vi "CreateTDMSFileExample_ForDataExplorer.vi"() -> ()   [LabVIEW 2017]
uses:
  <vilib>/addons/InsightCM/Utilities/Tdms/Tdms.lvlib
  <vilib>/addons/InsightCM/Utilities/GlobalConfiguration/GlobalConfiguration.lvlib
  <vilib>/measure/NI_MABase.lvlib
  <vilib>/addons/InsightCM/Utilities/DeviceModelHelpers/DeviceModelHelpers.lvlib
panel:
  out "Created TDMS Files":path[](array[path])
  # "Run this VI and inspect the file(s) below"
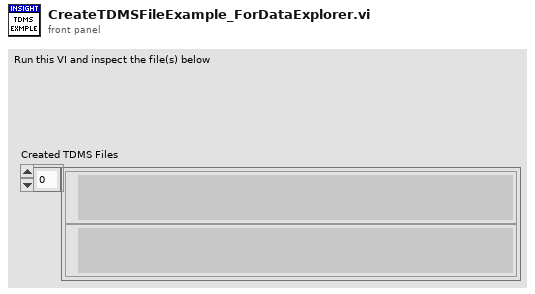
[diagram p1: front panel]
types:
  T1 = typedef "R2_DeviceModel.ctl" = cluster{"Device":T2, "Channels":T10[], "Tags":T12[]}
  T2 = typedef "R2_Device.ctl" = cluster{"Id":string, "Name":string, "DeviceType":string, "HardwareName":string, "IpAddress":string, "HardwareInfo":T3[], "ApplicationType":string, "ApplicationVersion":string, "EquipmentIds":string[], "ConfigurationVersion":string, "State":T4, "Properties":T3[], "DataGroups":T5[], "BurstModeTrigger":T9}
  T3 = typedef "KeyValuePair.ctl" = cluster{"Key":string, "Value":string}
  T4 = typedef "DeviceState.ctl" = cluster{"Disabled":bool}
  T5 = typedef "R2_DataGroup.ctl" = cluster{"Name":string, "OperatingStates":T6[], "Properties":T3[], "EquipmentIds":string[], "AssetNodeId":string}
  T6 = typedef "OperatingState.ctl" = cluster{"Name":string, "Properties":T3[], "Triggers":T7[]}
  T7 = typedef "Trigger.ctl" = cluster{"Type":string, "Expression":string, "Conditions":T8[]}
  T8 = typedef "Condition.ctl" = cluster{"Source":string, "Type":string, "Operator":string, "CompareTo":string, "DwellSeconds":dbl}
  T9 = typedef "BurstModeTrigger.ctl" = cluster{"Trigger":T7, "SampleRate":string, "AcquisitionLength":string}
  T10 = typedef "R2_Channel.ctl" = cluster{"Id":string, "DeviceId":string, "Name":string, "ChannelType":string, "HardwareKey":string, "HardwareChannel":string, "DataGroup":string, "Keywords":string[], "EquipmentIds":string[], "Properties":T3[], "Metrics":T11[], "AssetNodeId":string, "MeasType":string, "AssetName":string}
  T11 = typedef "Metric.ctl" = cluster{"Id":string, "Name":string, "Unit":string, "Properties":T3[], "MetricDefinitionInstanceId":string}
  T12 = typedef "Tag.ctl" = cluster{"Id":string, "Path":string, "Name":string, "Datatype":string, "Props":T3[], "Keywords":string[]}
  T13 = typedef "Equipment.ctl" = cluster{"Id":string, "ParentId":string, "Levelname":string, "Name":string, "Properties":T3[]}
  T14 = enum16{"open", "open or create", "create or replace", "create", "open (read-only)"}
  T15 = typedef "Tdms.lvlib/Property.ctl" = cluster{"Name":string, "Value":variant}
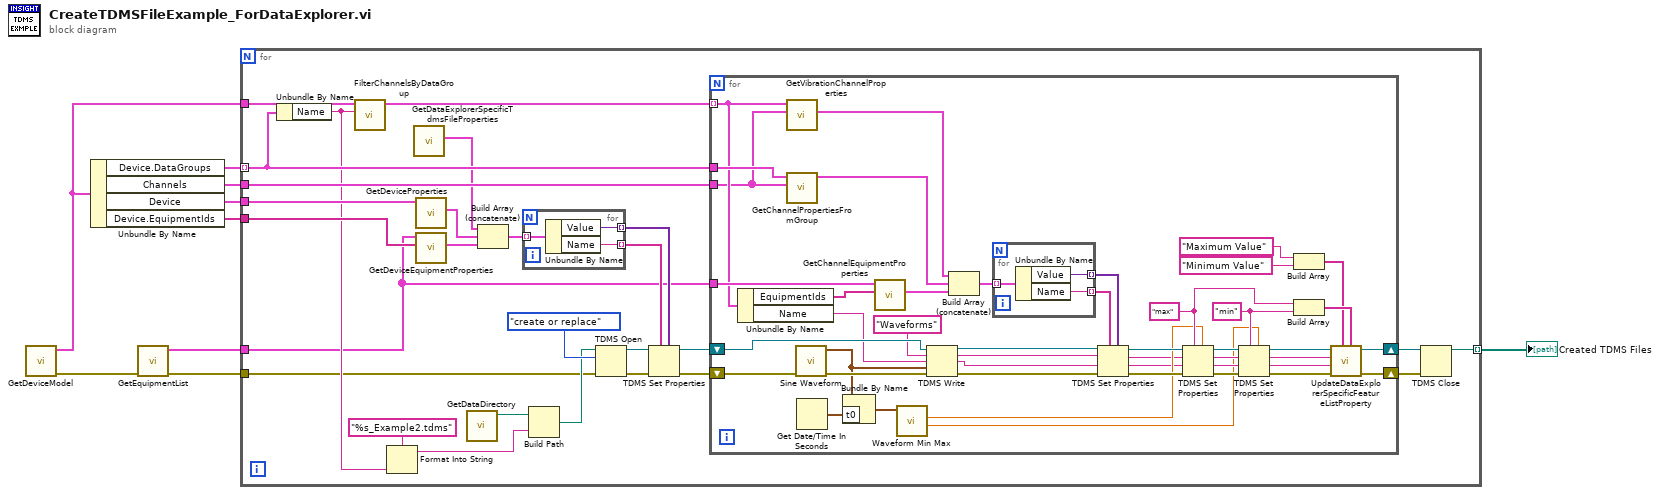
[diagram p0: block diagram]
diagram:
  n1 = call <vilib>:"GetDeviceModel.vi"() -> ("error out"=w3:errorcluster, "device model"=w5:T1)  [unwired: 9 in, 1 out]
  n2 = Unbundle By Name(w5) -> ("Device.DataGroups"=w6:T5[], "Channels"=w7:T10[], "Device"=w9:T2, "Device.EquipmentIds"=w8:string[])
  n3 = call <vilib>:"GetEquipmentList.vi"("error in (no error)"=w3) -> ("error out"=w2:errorcluster, "equipment list"=w1:T13[])  [unwired: 8 in, 1 out]
  n4 = for {
    tunnel: w2 -> [w11]
    tunnel: w9 -> [w36]
    tunnel: w8 -> [w35]
    tunnel: w7 -> [w21]
    tunnel: w6 -> [w17] mode=indexing
    tunnel: w5 -> [w19]
    tunnel: [w13] -> w4 mode=indexing
    tunnel: w1 -> [w10]
    n5 = Unbundle By Name(w17) -> ("Name"=w15:string)
    n6 = call <vilib>:"FilterChannelsByDataGroup.vi"("group"=w15, "device model"=w19) -> ("channels in data group"=w20:T10[])  [unwired: 8 in, 1 out]
    n7 = Format Into String(format string="%s_Example2.tdms", w15) -> (resulting string=w14:string)  [unwired: 2 in, 1 out]
    n8 = call <vilib>:"GetDataExplorerSpecificTdmsFileProperties.vi"() -> ("TDMS properties"=w12:T15[])  [unwired: 10 in, 1 out]
    n9 = call <vilib>:"GetDeviceProperties.vi"("device"=w36) -> ("tdms properties"=w31:T15[])  [unwired: 10 in]
    n10 = call <vilib>:"GetDeviceEquipmentProperties.vi"("equipment Ids"=w35, "equipment list"=w10) -> ("tdms properties"=w30:T15[])  [unwired: 9 in]
    n11 = call <vilib>:"GetDataDirectory.vi"() -> ("data directory"=w22:path)  [unwired: 10 in, 1 out]
    n12 = Build Array (concatenate)(w12, w31, w30) -> (w29:T15[])
    n13 = for {
      tunnel: w29 -> [w87] mode=indexing
      tunnel: [w86] -> w28 mode=indexing
      tunnel: [w85] -> w27 mode=indexing
      n14 = Unbundle By Name(w87) -> ("Value"=w85:variant, "Name"=w86:string)
    }
    n15 = Build Path(base path=w22, name or relative path=w14) -> (appended path=w18:path)
    n16 = TDMS Open(8:w11, 10:T14."create or replace" ("operation (0:open)"), 11:w18) -> (0:w32:errorcluster, 3:w33:refnum<k34>)  [unwired: 4 in]
    n17 = TDMS Set Properties(5:w27, 7:w28, 8:w32, 11:w33) -> (0:w26:errorcluster, 3:w25:refnum<k34>)  [unwired: 2 in, 2 out]
    n18 = for {
      shift-right: [w46] -> w23
      shift-left: w26 -> [w72]
      tunnel: w21 -> [w64]
      tunnel: w10 -> [w80]
      shift-right: [w45] -> w24
      shift-left: w25 -> [w74]
      tunnel: w20 -> [w65] mode=indexing
      tunnel: w17 -> [w66]
      w52 = "min" ("property names")
      w53 = "max" ("property names")
      n19 = Unbundle By Name(w65) -> ("EquipmentIds"=w81:string[], "Name"=w70:string)
      n20 = call <vilib>:"GetVibrationChannelProperties.vi"("all channels"=w64, "channel"=w65) -> ("TDMS properties"=w62:T15[])  [unwired: 9 in]
      n21 = call <vilib>:"GetChannelPropertiesFromGroup.vi"("all channels"=w64, "group"=w66) -> ("tdms properties"=w63:T15[])  [unwired: 9 in]
      n22 = call <vilib>:"Sine Waveform.vi"("error in (no error)"=w72) -> ("error out"=w71:errorcluster, "signal out"=w39:waveform(dbl))  [unwired: 9 in]
      n23 = Get Date/Time In Seconds() -> (seconds since 1Jan1904=w37:timestamp)
      n24 = Bundle By Name(cluster=w39, "t0"=w37) -> (w38:waveform(dbl))
      n25 = call <vilib>:"GetChannelEquipmentProperties.vi"("equipment Ids"=w81, "equipment list"=w80) -> ("TDMS properties"=w79:T15[])  [unwired: 9 in]
      n26 = call <vilib>:"Waveform Min Max.vi"("waveform in"=w38) -> ("Y min"=w42:dbl, "Y max"=w43:dbl)  [unwired: 5 in, 4 out]
      n27 = TDMS Write(0:w74, 5:"Waveforms" ("group name in (Untitled)"), 7:w70, 9:w39, 11:w71) -> (4:w73:refnum<k34>, 6:w68:string, 8:w67:string, 15:w75:errorcluster)  [unwired: 1 in]
      n28 = Build Array (concatenate)(w62, w63, w79) -> (w78:T15[])
      n29 = for {
        tunnel: w78 -> [w84] mode=indexing
        tunnel: [w83] -> w77 mode=indexing
        tunnel: [w82] -> w76 mode=indexing
        n30 = Unbundle By Name(w84) -> ("Value"=w82:variant, "Name"=w83:string)
      }
      n31 = TDMS Set Properties(5:w76, 7:w77, 8:w75, 9:w67, 10:w68, 11:w73) -> (0:w47:errorcluster, 1:w40:string, 2:w41:string, 3:w44:refnum<k34>)
      n32 = TDMS Set Properties(5:w43, 7:w53, 8:w47, 9:w40, 10:w41, 11:w44) -> (0:w60:errorcluster, 1:w56:string, 2:w57:string, 3:w61:refnum<k34>)
      n33 = TDMS Set Properties(5:w42, 7:w52, 8:w60, 9:w56, 10:w57, 11:w61) -> (0:w59:errorcluster, 1:w55:string, 2:w58:string, 3:w54:refnum<k34>)
      n34 = Build Array("Maximum Value" ("property names"), "Minimum Value" ("property names")) -> (w48:string[])
      n35 = Build Array(w53, w52) -> (w51:string[])
      n36 = call <vilib>:"UpdateDataExplorerSpecificFeatureListProperty.vi"("features"=w51, "display names"=w48, "error in (no error)"=w59, "channel"=w55, "group"=w58, "TDMS ref in"=w54) -> ("error out"=w46:errorcluster, "TDMS ref out"=w45:refnum<k34>)  [unwired: 2 in, 2 out]
    }
    n37 = TDMS Close(8:w23, 11:w24) -> (3:w13:path)  [unwired: 1 out]
  }
  "Created TDMS Files" <- w4
